vi "Thev-Process Response.vi"(0 "State in":T1, 5 "Params":T5 {"LProbe" items=["None"=-1, "Probe A"=0, "Probe B"=1]; "Rprobe" items=["None"=-1, "Probe A"=0, "Probe B"=1]}, 7 "Path":path) -> (4 "State out":T1, 15 "error out":errorcluster)   [LabVIEW 2015]
uses:
  Typedefs/Thev-Parameters.ctl
  Typedefs/Thev-Stimulus.ctl
  Typedefs/Thev-Find.ctl
  Misc VIs/Equipment Control/ER10X/ER10X-Probe.ctl
  Typedefs/Thev-Optimization Parameters.ctl
  Typedefs/Thev-State.ctl
  D:/Experiment VIs/Misc VIs/Equipment Control/ER10X/ER10XConnect.NET.dll
  Misc VIs/Equipment Control/ER10X/ER10XConnect.NET.dll
  Typedefs/Thev-Procedure Phase.ctl
  Typedefs/Thev-Progress Table Element.ctl
  Typedefs/Thev-Optimization Result.ctl
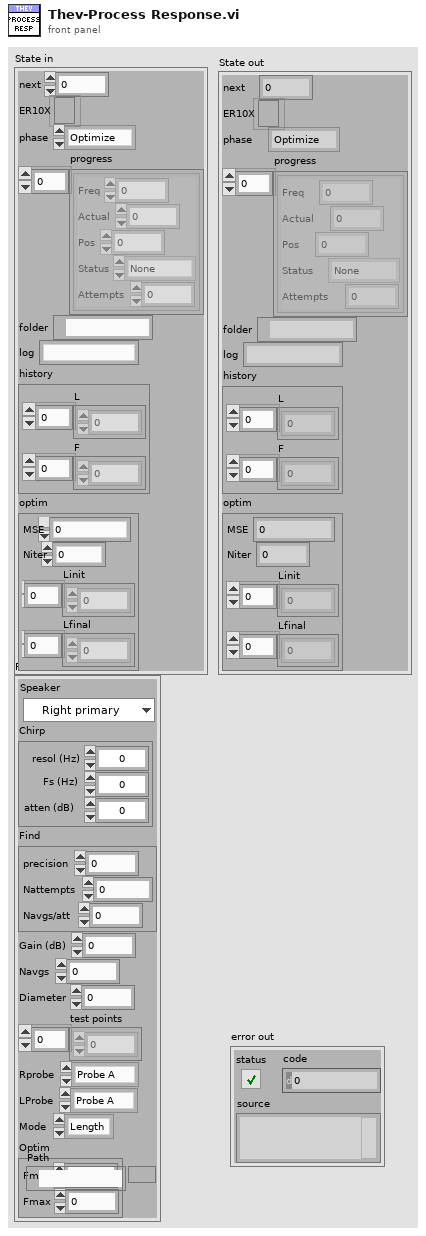
[diagram p1: front panel]
types:
  T1 = typedef "Thev-State.ctl" = cluster{"next":i32, "ER10X":refnum<k24>, "phase":T2, "progress":T3[], "folder":path, "log":string, "history":cluster{"L":dbl[], "F":dbl[]}, "optim":T4}
  T2 = typedef "Thev-Procedure Phase.ctl" = enum16{"Optimize", "Measure", "Compute", "Finished"}
  T3 = typedef "Thev-Progress Table Element.ctl" = cluster{"Freq":dbl, "Actual":dbl, "Pos":dbl, "Status":enum16{"None", "Measuring", "Finished"}, "Attempts":i32}
  T4 = typedef "Thev-Optimization Result.ctl" = cluster{"MSE":dbl, "Niter":i32, "Linit":dbl[], "Lfinal":dbl[]}
  T5 = typedef "Thev-Parameters.ctl" = cluster{"Speaker":enum16{"Right primary", "Right secondary", "Left primary", "Left secondary"}, "Chirp":T6, "Find":T7, "Gain (dB)":dbl, "Navgs":i32, "Diameter":dbl, "test points":dbl[], "Rprobe":T8, "LProbe":T8, "Mode":enum16{"Length", "Freq"}, "Optim":T9}
  T6 = typedef "Thev-Stimulus.ctl" = cluster{"resol (Hz)":dbl, "atten (dB)":dbl, "Fs (Hz)":dbl}
  T7 = typedef "Thev-Find.ctl" = cluster{"precision":dbl, "Nattempts":i32, "Navgs/att":i32}
  T8 = typedef "ER10X-Probe.ctl" = i32
  T9 = typedef "Thev-Optimization Parameters.ctl" = cluster{"Fmin":dbl, "Fmax":dbl}
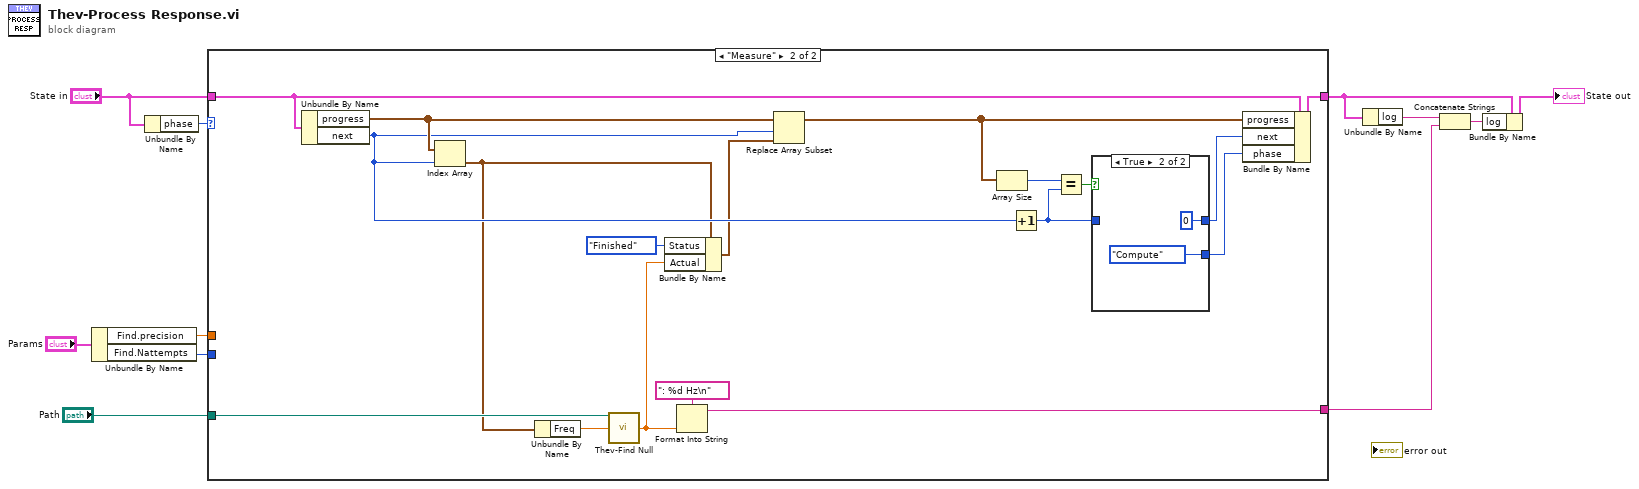
[diagram p0: block diagram]
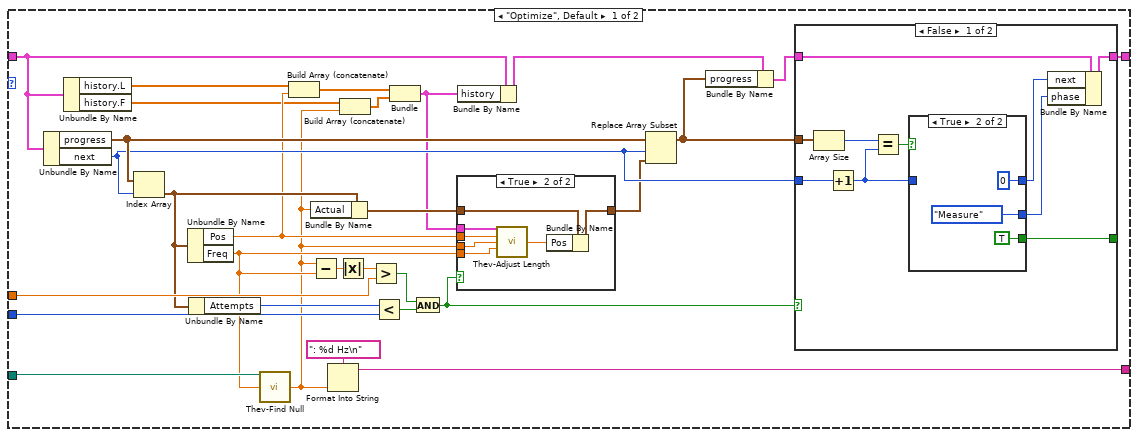
[diagram p2: hidden frame]
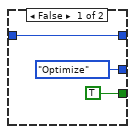
[diagram p3: hidden frame]
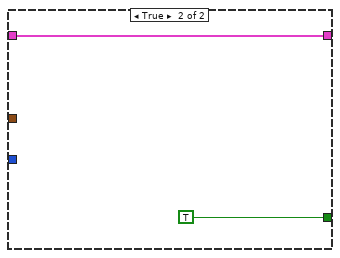
[diagram p4: hidden frame]
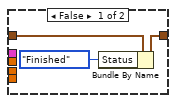
[diagram p5: hidden frame]
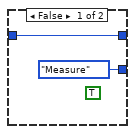
[diagram p6: hidden frame]
diagram:
  n1 = Unbundle By Name("Params") -> ("Find.precision"=w2:dbl, "Find.Nattempts"=w1:i32)
  n2 = Unbundle By Name("State in") -> ("phase"=w11:T2)
  n3 = case shown="\"Measure\"" w11 {
    tunnel: "Path" -> [w40 w73]
    tunnel: [w38 w69] -> w8
    tunnel: "State in" -> [w23 w80]
    tunnel: [w16 w86] -> w4
    tunnel: w2 -> [w32 _]
    tunnel: w1 -> [w29 _]
    frame "Optimize", Default {
      n4 = Unbundle By Name(w23) -> ("progress"=w37:T3[], "next"=w36:i32)
      n5 = Unbundle By Name(w23) -> ("history.L"=w22:dbl[], "history.F"=w20:dbl[])
      n6 = Index Array(array=w37, index=w36) -> (element=w28:T3)
      n7 = Unbundle By Name(w28) -> ("Pos"=w21:dbl, "Freq"=w24:dbl)
      n8 = Unbundle By Name(w28) -> ("Attempts"=w27:i32)
      n9 = call "Thev-Find Null.vi"("Path"=w40, "Freq"=w24) -> ("Null freq (Hz)"=w19:dbl)  [unwired: 12 in, 1 out]
      n10 = Build Array (concatenate)(w22, w21) -> (w14:dbl[])
      n11 = Bundle By Name(cluster=w28, "Actual"=w19) -> (w26:T3)
      n12 = Subtract(x=w19, y=w24) -> (x-y=w34:dbl)
      n13 = Format Into String(format string=": %d Hz\n", w19) -> (resulting string=w38:string)  [unwired: 2 in, 1 out]
      n14 = Absolute Value(x=w34) -> (abs(x)=w33:dbl)
      n15 = Build Array (concatenate)(w20, w19) -> (w13:dbl[])
      n16 = Greater?(x=w33, y=w32) -> (0:w31:bool)
      n17 = Less?(x=w27, y=w29) -> (x < y?=w30:bool)
      n18 = Bundle(w14, w13) -> (w12:cluster{dbl[], dbl[]})  [unwired: 1 in]
      n19 = And(x=w31, y=w30) -> (x .and. y?=w18:bool)
      n20 = case shown="True" w18 {
        tunnel: w26 -> [w61 w65]
        tunnel: [w60 w63] -> w25
        tunnel: w19 -> [_ w67]
        tunnel: w24 -> [_ w66]
        tunnel: w21 -> [_ w68]
        tunnel: w12 -> [_ w64]
        frame False {
          n21 = Bundle By Name(cluster=w61, "Status"=enum16{"None", "Measuring", "Finished"}."Finished") -> (w60:T3)
        }
        frame True {
          n22 = call "Thev-Adjust Length.vi"("history"=w64, "Pos"=w68, "Actual"=w67, "Freq"=w66) -> ("Pos out"=w62:dbl)  [unwired: 11 in]
          n23 = Bundle By Name(cluster=w65, "Pos"=w62) -> (w63:T3)
        }
      }
      n24 = Bundle By Name(cluster=w23, "history"=w12) -> (w15:T1)
      n25 = Replace Array Subset(array=w37, new element=w25, index=w36) -> (w35:T3[])
      n26 = Bundle By Name(cluster=w15, "progress"=w35) -> (w17:T1)
      n27 = case shown="False" w18 {
        tunnel: w36 -> [w50 _]
        tunnel: w35 -> [w49 _]
        tunnel: [w45 TRUE] -> _
        tunnel: w17 -> [w44 w57]
        tunnel: [w43 w57] -> w16
        frame False {
          n28 = Array Size(array=w49) -> (size(s)=w48:i32)
          n29 = Increment(x=w50) -> (x+1=w46:i32)
          n30 = Equal?(x=w48, y=w46) -> (x = y?=w47:bool)
          n31 = case shown="True" w47 {
            tunnel: [Thev-Procedure_Phase."Optimize" ("phase") Thev-Procedure_Phase."Measure" ("phase")] -> w41
            tunnel: [w53 0] -> w42
            tunnel: w46 -> [w53 _]
            tunnel: [TRUE TRUE] -> w45
            frame False {
            }
            frame True {
            }
          }
          n32 = Bundle By Name(cluster=w44, "next"=w42, "phase"=w41) -> (w43:T1)
        }
        frame True {
        }
      }
    }
    frame "Measure" {
      n33 = Unbundle By Name(w80) -> ("progress"=w78:T3[], "next"=w77:i32)
      n34 = Index Array(array=w78, index=w77) -> (element=w71:T3)
      n35 = Unbundle By Name(w71) -> ("Freq"=w70:dbl)
      n36 = call "Thev-Find Null.vi"("Path"=w73, "Freq"=w70) -> ("Null freq (Hz)"=w72:dbl)  [unwired: 12 in, 1 out]
      n37 = Bundle By Name(cluster=w71, "Status"=enum16{"None", "Measuring", "Finished"}."Finished", "Actual"=w72) -> (w76:T3)
      n38 = Format Into String(format string=": %d Hz\n", w72) -> (resulting string=w69:string)  [unwired: 2 in, 1 out]
      n39 = Replace Array Subset(array=w78, new element=w76, index=w77) -> (w75:T3[])
      n40 = Array Size(array=w75) -> (size(s)=w85:i32)
      n41 = Increment(x=w77) -> (x+1=w83:i32)
      n42 = Equal?(x=w85, y=w83) -> (x = y?=w84:bool)
      n43 = case shown="True" w84 {
        tunnel: [Thev-Procedure_Phase."Measure" ("phase") Thev-Procedure_Phase."Compute" ("phase")] -> w81
        tunnel: [w88 0] -> w82
        tunnel: w83 -> [w88 _]
        frame False {
          (unwired) TRUE
        }
        frame True {
        }
      }
      n44 = Bundle By Name(cluster=w80, "progress"=w75, "next"=w82, "phase"=w81) -> (w86:T1)
    }
  }
  n45 = Unbundle By Name(w4) -> ("log"=w9:string)
  n46 = Concatenate Strings(w9, w8) -> (w6:string)
  n47 = Bundle By Name(cluster=w4, "log"=w6) -> (→"State out":T1)
